vi "Field Get Fields from List.vi"(8 "error in (no error)":errorcluster, 10 "sxFieldIdsCSV (\"\")":string, 11 "Connection Refnum":T4) -> (0 "error out":errorcluster, 1 "new Fields CSV":string, 2 "Fields":T1[](array[typedef]), 3 "Connection Refnum":T4)   [LabVIEW 2011]
uses:
  SI.LIB/ODBC/SQL Controls/Connection Refnum.ctl
  Field Record.ctl
  Field DataTypes.ctl
  Field NextItem.ctl
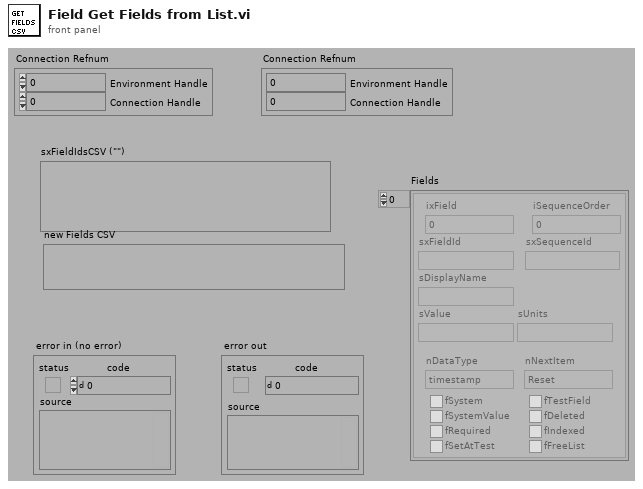
[diagram p1: front panel]
types:
  T1 = typedef "Field Record.ctl" = cluster{"ixField":i32, "iSequenceOrder":i32, "sxFieldId":string, "sxSequenceId":string, "sDisplayName":string, "sValue":string, "sUnits":string, "nDataType":T2, "nNextItem":T3, "fSystem":bool, "fSystemValue":bool, "fRequired":bool, "fSetAtTest":bool, "fTestField":bool, "fDeleted":bool, "fIndexed":bool, "fFreeList":bool}
  T2 = typedef "Field DataTypes.ctl" = enum32{"text", "numeric", "list", "timestamp", "boolean"}
  T3 = typedef "Field NextItem.ctl" = enum32{"Reset", "Retain", "Auto-Increment"}
  T4 = typedef "Connection Refnum.ctl" = cluster{"Environment Handle":i32, "Connection Handle":i32}
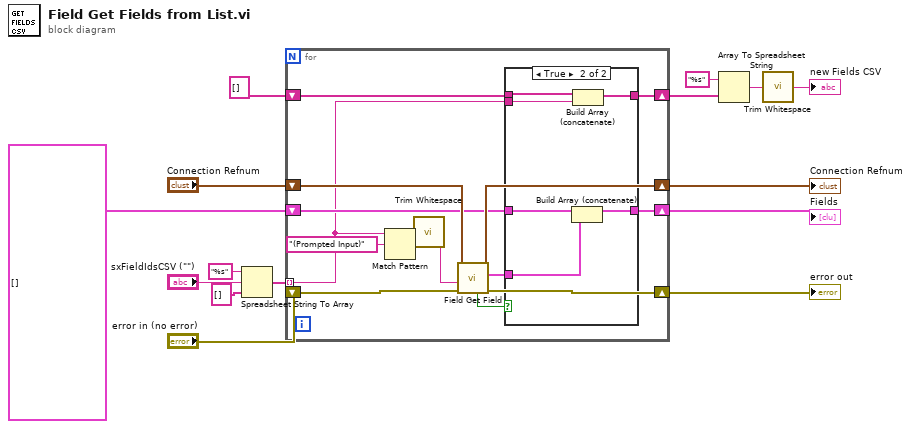
[diagram p0: block diagram]
diagram:
  n1 = Spreadsheet String To Array(format string="%s", spreadsheet string="sxFieldIdsCSV (\"\")", array type (2D Dbl)=string[] []) -> (array=w1:string[])  [unwired: 1 out]
  n2 = for {
    shift-right: [w28] -> w11
    shift-left: "error in (no error)" -> [w29]
    tunnel: w1 -> [w16] mode=indexing
    shift-right: [w26] -> w12
    shift-left: "Connection Refnum" -> [w27]
    shift-right: [w22] -> w10
    shift-left: T1[] [] -> [w24]
    shift-right: [w20] -> w6
    shift-left: string[] [] -> [w21]
    n3 = Match Pattern(string=w16, regular expression="(Prompted Input)") -> (before substring=w18:string)  [unwired: 1 in, 3 out]
    n4 = call <vilib>:"Trim Whitespace.vi"("string"=w18) -> ("trimmed string"=w17:string)  [unwired: 1 in]
    n5 = call "Field Get Field.vi"("error in (no error)"=w29, "sFieldId or sDisplayName (\"\")"=w17, "Connection Refnum"=w27) -> ("error out"=w28:errorcluster, "Field"=w23:T1, "Connection Refnum"=w26:T4, "Data Present?"=w25:bool)  [unwired: 2 in, 3 out]
    n6 = case shown="True" w25 {
      tunnel: w24 -> [w31 w37]
      tunnel: w23 -> [_ w36]
      tunnel: [w31 w35] -> w22
      tunnel: w21 -> [w30 w34]
      tunnel: [w30 w33] -> w20
      tunnel: w16 -> [_ w32]
      frame False {
      }
      frame True {
        n7 = Build Array (concatenate)(w37, w36) -> (w35:T1[])
        n8 = Build Array (concatenate)(w34, w32) -> (w33:string[])
      }
    }
  }
  "error out" <- w11
  "Connection Refnum" <- w12
  "Fields" <- w10
  n9 = Array To Spreadsheet String(array=w6, 3:"%s" ("format string")) -> (spreadsheet string=w7:string)  [unwired: 1 out]
  n10 = call <vilib>:"Trim Whitespace.vi"("string"=w7) -> ("trimmed string"=→"new Fields CSV":string)  [unwired: 1 in]
